vi "Untitled 1 (SubVI).vi"() -> ()   [LabVIEW 2019]
panel:
  out "Numeric 2":i32=1
  out "Numeric":i32
  in  "stop":bool
  out "linkermotor : d":dbl=0.4
  out "rechtermotor : d":dbl=0.4
  out "linkermotor :  r":dbl=0.4
  out "rechtermotor : r":dbl
  out "linkermotor : l":dbl=0.4
  out "rechtermotor : l":dbl
  in  "de universele stop":bool
  in  "String":string
  in  "OK Button":bool
  # "l :  linksafslaan\nr : rechtsaflsaan\nd : rechtdoorgaan"
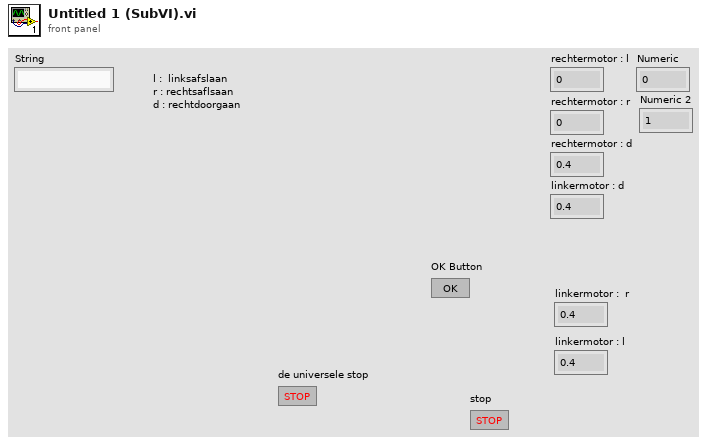
[diagram p1: front panel]
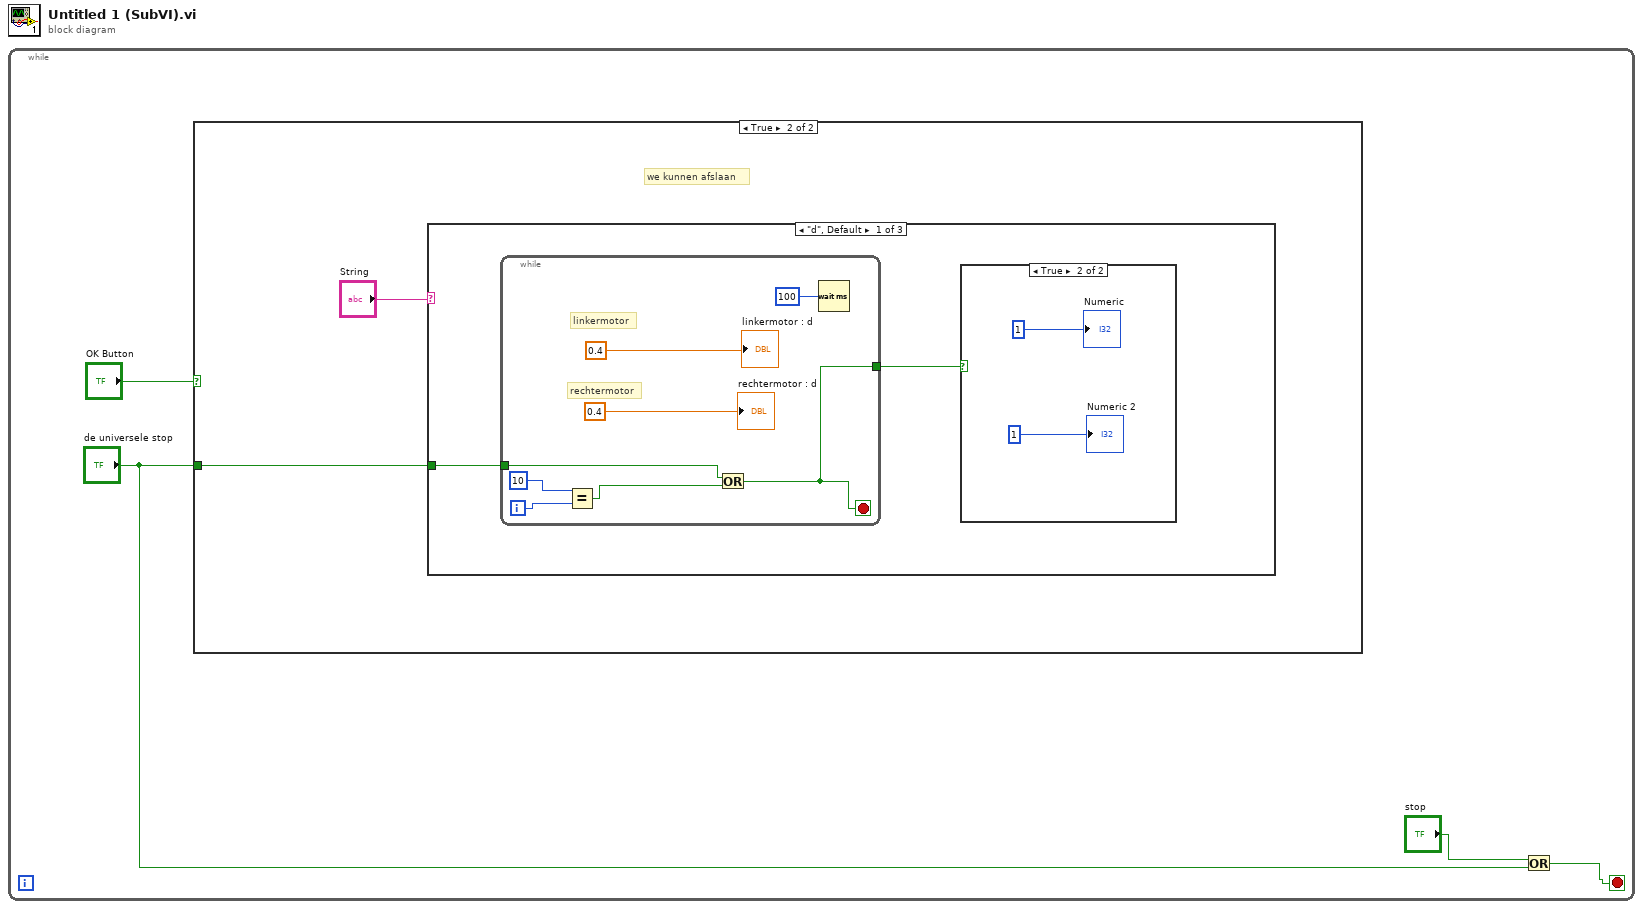
[diagram p0: block diagram]
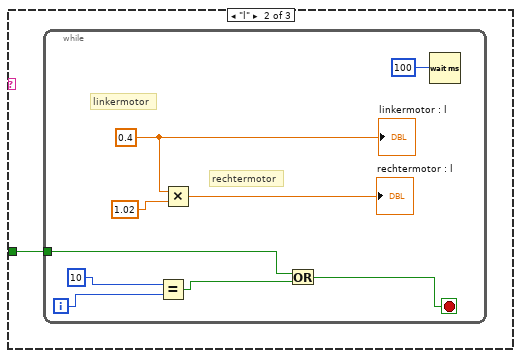
[diagram p4: hidden frame]
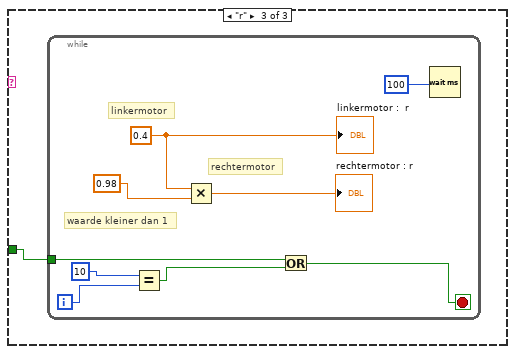
[diagram p5: hidden frame]
diagram:
  n1 = while {
    stop <- w3 stop-if-true
    n2 = case shown="True" "OK Button" {
      tunnel: "de universele stop" -> [_ w5]
      frame False {
      }
      frame True {
        # "we kunnen afslaan"
        n3 = case shown="\"d\", Default" "String" {
          tunnel: w5 -> [w8 w19 w29]
          frame "d", Default {
            n4 = while {
              tunnel: w8 -> [w15]
              tunnel: [w11] -> w7
              i -> [w17]
              stop <- w11 stop-if-true
              # "rechtermotor"
              # "linkermotor"
              n5 = Equal?(x=10, y=w17) -> (x = y?=w16:bool)
              n6 = Or(x=w15, y=w16) -> (x .or. y?=w11:bool)
              n7 = Wait (ms)(milliseconds to wait=100) -> ()  [unwired: 1 out]
              "rechtermotor : d" <- 0.4
              "linkermotor : d" <- 0.4
            }
            n8 = case shown="True" w7 {
              frame False {
              }
              frame True {
                "Numeric" <- 1
                "Numeric 2" <- 1
              }
            }
          }
          frame "l" {
            n9 = while {
              tunnel: w19 -> [w23]
              i -> [w26]
              stop <- w24 stop-if-true
              w28 = 0.4
              # "rechtermotor"
              # "linkermotor"
              n10 = Equal?(x=10, y=w26) -> (x = y?=w25:bool)
              n11 = Multiply(x=w28, y=1.02) -> (x*y=→"rechtermotor : l":dbl)
              n12 = Or(x=w23, y=w25) -> (x .or. y?=w24:bool)
              n13 = Wait (ms)(milliseconds to wait=100) -> ()  [unwired: 1 out]
              "linkermotor : l" <- w28
            }
          }
          frame "r" {
            n14 = while {
              tunnel: w29 -> [w32]
              i -> [w35]
              stop <- w34 stop-if-true
              w38 = 0.4
              # "waarde kleiner dan 1"
              # "rechtermotor"
              # "linkermotor"
              n15 = Equal?(x=10, y=w35) -> (x = y?=w33:bool)
              n16 = Multiply(x=w38, y=0.98) -> (x*y=→"rechtermotor : r":dbl)
              n17 = Or(x=w32, y=w33) -> (x .or. y?=w34:bool)
              n18 = Wait (ms)(milliseconds to wait=100) -> ()  [unwired: 1 out]
              "linkermotor :  r" <- w38
            }
          }
        }
      }
    }
    n19 = Or(x="stop", y="de universele stop") -> (x .or. y?=w3:bool)
  }
